vi "校准参数转data(子VI).vi"(10 "改变?":bool, 11 "校准信息":T1) -> (3 "数组":string[][](array[string]))   [LabVIEW 2016, in "数据传输系统-05.lvlib"]
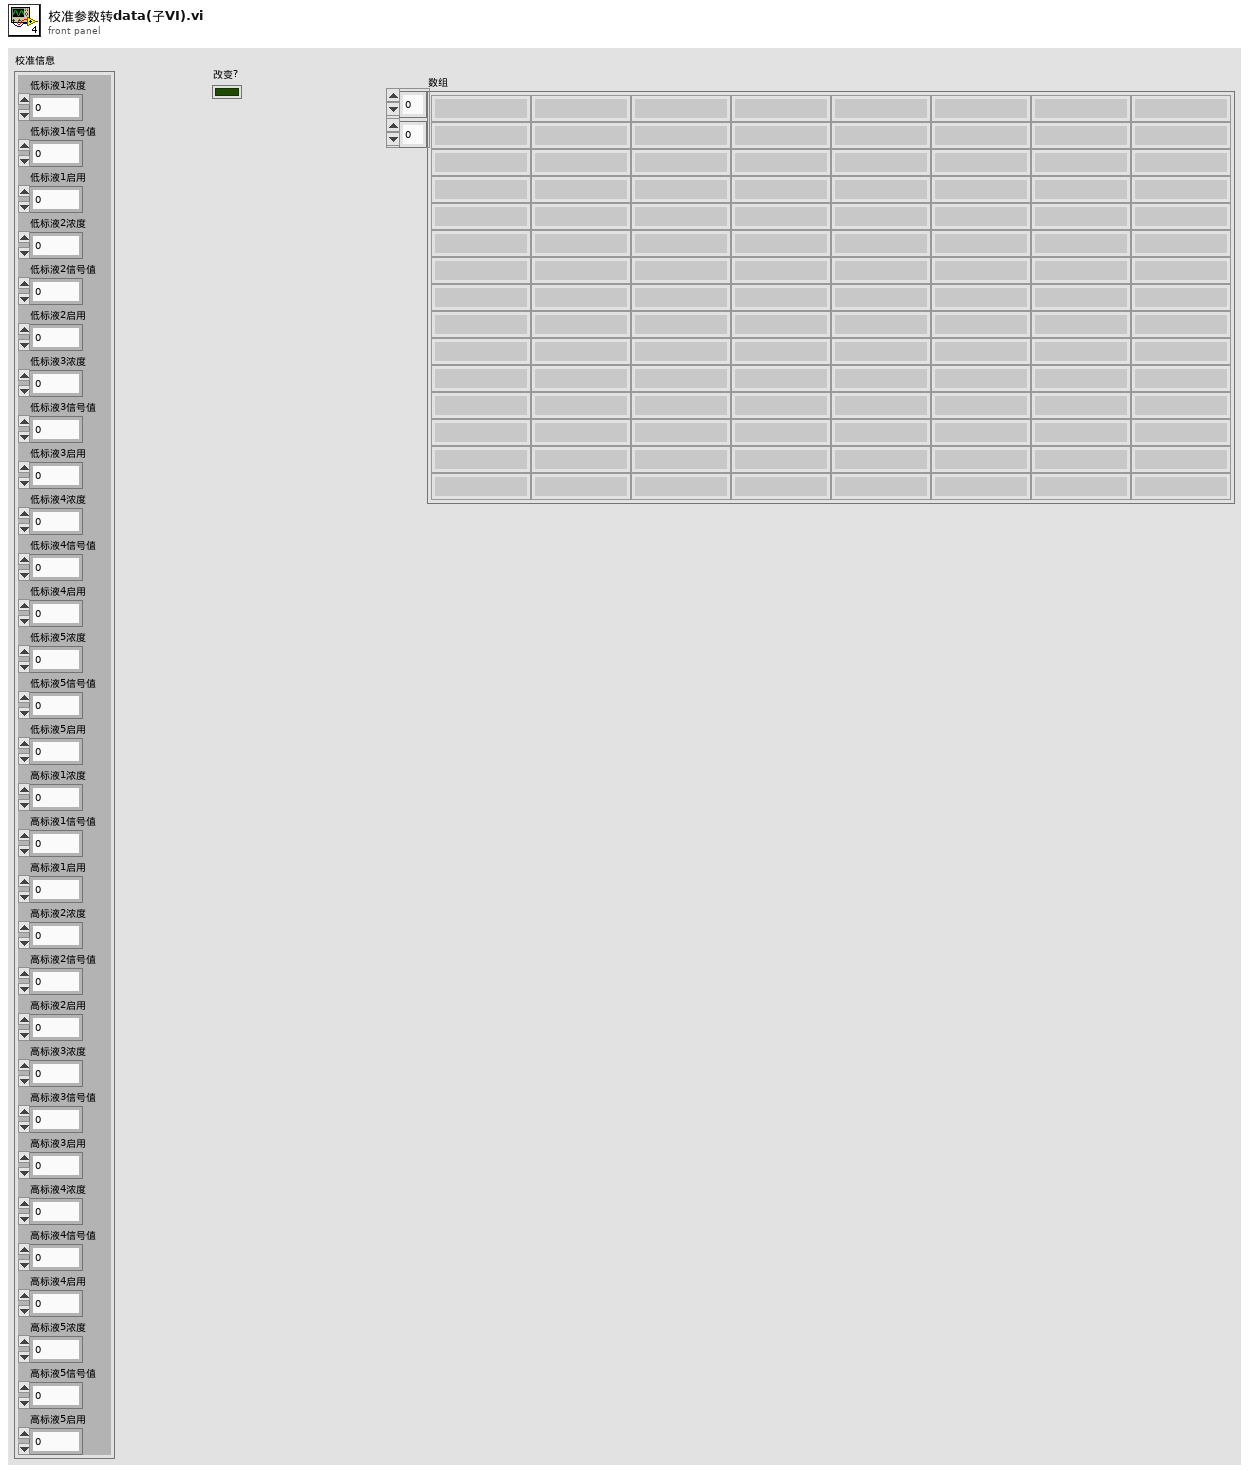
[diagram p1: front panel]
types:
  T1 = cluster{"低标液1浓度":dbl, "低标液1信号值":dbl, "低标液1启用":u16, "低标液2浓度":dbl, "低标液2信号值":dbl, "低标液2启用":u16, "低标液3浓度":dbl, "低标液3信号值":dbl, "低标液3启用":u16, "低标液4浓度":dbl, "低标液4信号值":dbl, "低标液4启用":u16, "低标液5浓度":dbl, "低标液5信号值":dbl, "低标液5启用":u16, "高标液1浓度":dbl, "高标液1信号值":dbl, "高标液1启用":u16, "高标液2浓度":dbl, "高标液2信号值":dbl, "高标液2启用":u16, "高标液3浓度":dbl, "高标液3信号值":dbl, "高标液3启用":u16, "高标液4浓度":dbl, "高标液4信号值":dbl, "高标液4启用":u16, "高标液5浓度":dbl, "高标液5信号值":dbl, "高标液5启用":u16}
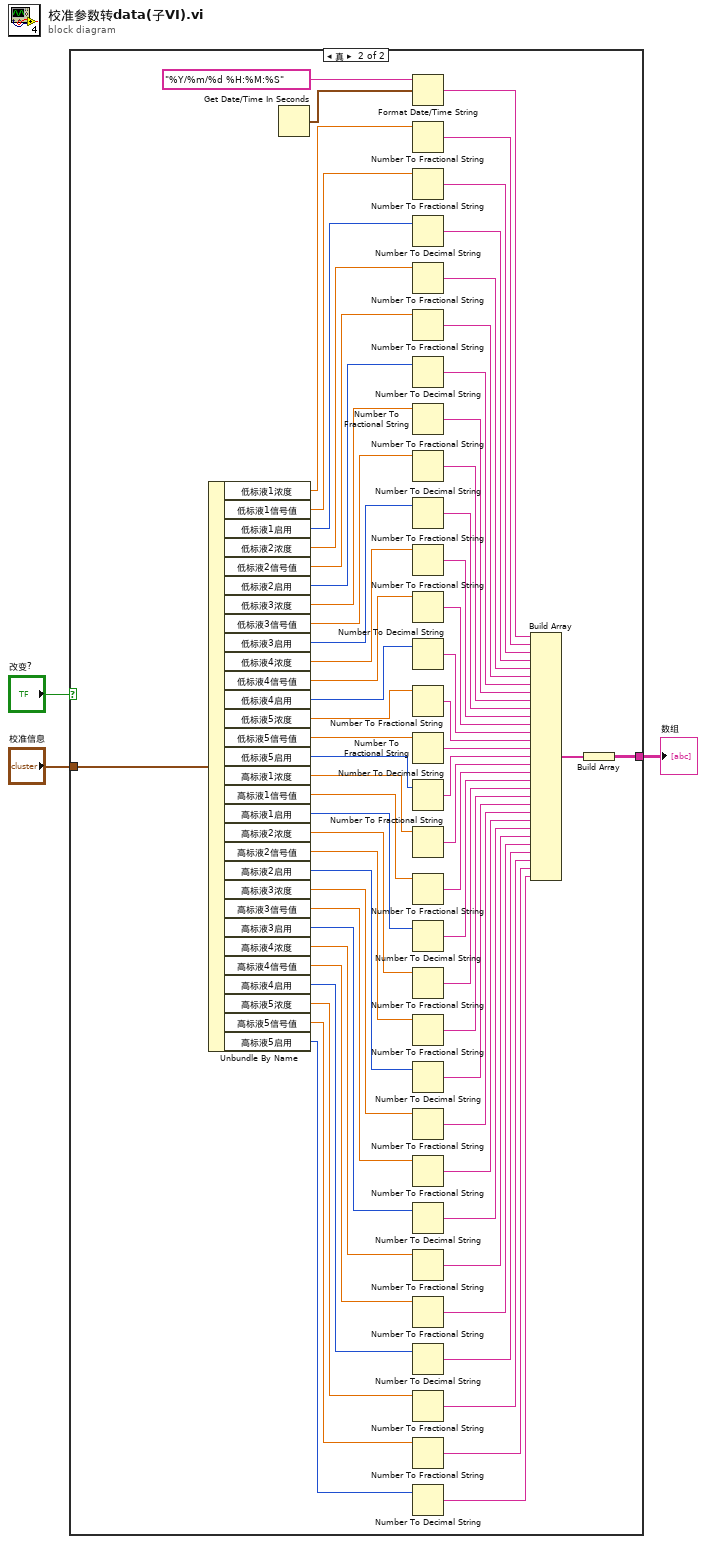
[diagram p0: block diagram]
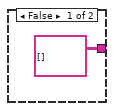
[diagram p2: hidden frame]
diagram:
  n1 = case shown="真" "改变?" {
    tunnel: [string[][] [] w70] -> w3
    tunnel: "校准信息" -> [_ w46]
    frame False {
    }
    frame True {
      n2 = Unbundle By Name(w46) -> ("低标液1浓度"=w47:dbl, "低标液1信号值"=w51:dbl, "低标液1启用"=w53:u16, "低标液2浓度"=w55:dbl, "低标液2信号值"=w57:dbl, "低标液2启用"=w44:u16, "低标液3浓度"=w59:dbl, "低标液3信号值"=w60:dbl, "低标液3启用"=w42:u16, "低标液4浓度"=w61:dbl, "低标液4信号值"=w62:dbl, "低标液4启用"=w40:u16, "低标液5浓度"=w38:dbl, "低标液5信号值"=w63:dbl, "低标液5启用"=w36:u16, "高标液1浓度"=w34:dbl, "高标液1信号值"=w33:dbl, "高标液1启用"=w32:u16, "高标液2浓度"=w28:dbl, "高标液2信号值"=w27:dbl, "高标液2启用"=w26:u16, "高标液3浓度"=w22:dbl, "高标液3信号值"=w21:dbl, "高标液3启用"=w20:u16, "高标液4浓度"=w19:dbl, "高标液4信号值"=w18:dbl, "高标液4启用"=w17:u16, "高标液5浓度"=w16:dbl, "高标液5信号值"=w15:dbl, "高标液5启用"=w14:u16)
      n3 = Get Date/Time In Seconds() -> (seconds since 1Jan1904=w49:timestamp)
      n4 = Format Date/Time String(time format string (%c)="%Y/%m/%d %H:%M:%S" ("时间格式字符串(%c)"), seconds (now)=w49) -> (date/time string=w45:string)  [unwired: 1 in]
      n5 = Number To Fractional String(number=w47) -> (F-format string=w50:string)  [unwired: 3 in]
      n6 = Number To Fractional String(number=w51) -> (F-format string=w52:string)  [unwired: 3 in]
      n7 = Number To Decimal String(number=w53) -> (decimal integer string=w54:string)  [unwired: 1 in]
      n8 = Number To Fractional String(number=w55) -> (F-format string=w56:string)  [unwired: 3 in]
      n9 = Number To Fractional String(number=w57) -> (F-format string=w58:string)  [unwired: 3 in]
      n10 = Number To Decimal String(number=w44) -> (decimal integer string=w43:string)  [unwired: 1 in]
      n11 = Number To Fractional String(number=w59) -> (F-format string=w64:string)  [unwired: 3 in]
      n12 = Number To Fractional String(number=w60) -> (F-format string=w65:string)  [unwired: 3 in]
      n13 = Number To Decimal String(number=w42) -> (decimal integer string=w41:string)  [unwired: 1 in]
      n14 = Number To Fractional String(number=w61) -> (F-format string=w66:string)  [unwired: 3 in]
      n15 = Number To Fractional String(number=w62) -> (F-format string=w67:string)  [unwired: 3 in]
      n16 = Number To Decimal String(number=w40) -> (decimal integer string=w39:string)  [unwired: 1 in]
      n17 = Number To Fractional String(number=w38) -> (F-format string=w37:string)  [unwired: 3 in]
      n18 = Number To Fractional String(number=w63) -> (F-format string=w68:string)  [unwired: 3 in]
      n19 = Number To Decimal String(number=w36) -> (decimal integer string=w35:string)  [unwired: 1 in]
      n20 = Number To Fractional String(number=w34) -> (F-format string=w31:string)  [unwired: 3 in]
      n21 = Number To Fractional String(number=w33) -> (F-format string=w30:string)  [unwired: 3 in]
      n22 = Number To Decimal String(number=w32) -> (decimal integer string=w29:string)  [unwired: 1 in]
      n23 = Number To Fractional String(number=w28) -> (F-format string=w25:string)  [unwired: 3 in]
      n24 = Number To Fractional String(number=w27) -> (F-format string=w24:string)  [unwired: 3 in]
      n25 = Number To Decimal String(number=w26) -> (decimal integer string=w23:string)  [unwired: 1 in]
      n26 = Number To Fractional String(number=w22) -> (F-format string=w13:string)  [unwired: 3 in]
      n27 = Number To Fractional String(number=w21) -> (F-format string=w12:string)  [unwired: 3 in]
      n28 = Number To Decimal String(number=w20) -> (decimal integer string=w11:string)  [unwired: 1 in]
      n29 = Number To Fractional String(number=w19) -> (F-format string=w10:string)  [unwired: 3 in]
      n30 = Number To Fractional String(number=w18) -> (F-format string=w9:string)  [unwired: 3 in]
      n31 = Number To Decimal String(number=w17) -> (decimal integer string=w8:string)  [unwired: 1 in]
      n32 = Number To Fractional String(number=w16) -> (F-format string=w7:string)  [unwired: 3 in]
      n33 = Number To Fractional String(number=w15) -> (F-format string=w6:string)  [unwired: 3 in]
      n34 = Number To Decimal String(number=w14) -> (decimal integer string=w5:string)  [unwired: 1 in]
      n35 = Build Array(w45, w50, w52, w54, w56, w58, w43, w64, w65, w41, w66, w67, w39, w37, w68, w35, w31, w30, w29, w25, w24, w23, w13, w12, w11, w10, w9, w8, w7, w6, w5) -> (w69:string[])
      n36 = Build Array(w69) -> (w70:string[][])
    }
  }
  "数组" <- w3
